vi "Clear LabVIEW Errors.vi"(8 "error in (no error)":errorcluster, 11 "Alarm Handler Actor in":refnum<class "Alarm Handler Actor.lvclass">) -> (0 "error out":errorcluster, 3 "Alarm Handler Actor out":refnum<class "Alarm Handler Actor.lvclass">)   [LabVIEW 2015, in "Alarm Handler Actor.lvclass"]
uses:
  Alarm Handler Actor.lvclass
  Alarm Handler Actor.lvclass/Alarm Handler Actor.ctl
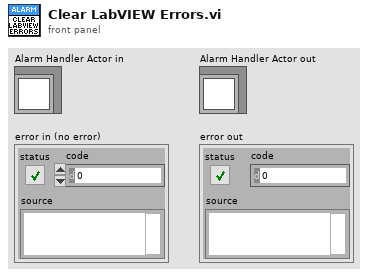
[diagram p1: front panel]
types:
  T1 = typedef "Alarm Handler Actor.lvclass/Active Alarm.ctl" = cluster{"Alarm Detail":T2, "Count":i32, "First Error":timestamp, "Last Error":timestamp, "LabVIEW Error":bool}
  T2 = typedef "Alarm Handler Actor.lvclass/Alarm Details.ctl" = cluster{"Code":i32, "Loop":i32, "Description":string, "Severity":i32, "Clear on Ack?":bool, "Log All Events?":bool}
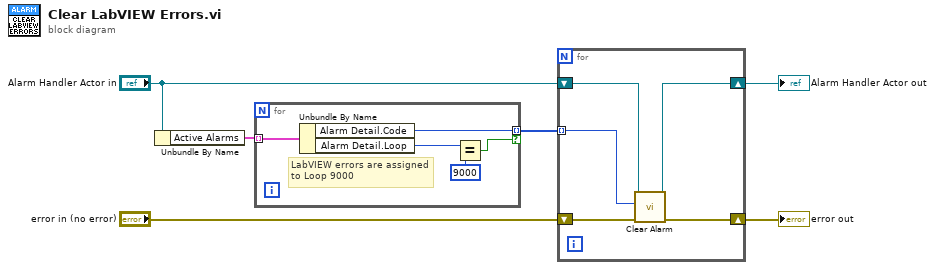
[diagram p0: block diagram]
diagram:
  n1 = Unbundle By Name("Alarm Handler Actor in") -> ("Active Alarms"=w4:T1[])
  n2 = for {
    tunnel: w4 -> [w11] mode=indexing
    tunnel: [w10] -> w6 mode=indexing if=w7
    # "LabVIEW errors are assigned to Loop 9000"
    n3 = Unbundle By Name(w11) -> ("Alarm Detail.Code"=w10:i32, "Alarm Detail.Loop"=w9:i32)
    n4 = Equal?(x=w9, y=9000 ("Element Data")) -> (x = y?=w7:bool)
  }
  n5 = for {
    shift-right: [w15] -> w2
    shift-left: "error in (no error)" -> [w14]
    shift-right: [w16] -> w1
    shift-left: "Alarm Handler Actor in" -> [w13]
    tunnel: w6 -> [w12] mode=indexing
    n6 = call "Clear Alarm.vi"("error in (no error)"=w14, "Alarm Code"=w12, "Alarm Handler Actor in"=w13) -> ("error out"=w15:errorcluster, "Alarm Handler Actor out"=w16:refnum<class "Alarm Handler Actor.lvclass">)  [unwired: 7 in]
  }
  "Alarm Handler Actor out" <- w1
  "error out" <- w2
